vi "Read_Input_1.vi"(8 "Error_In":errorcluster, 11 "Calculator_In":refnum<class "Calculator.lvclass">) -> (0 "Error_Out":errorcluster, 2 "Input_1":dbl, 3 "Calculator_Out":refnum<class "Calculator.lvclass">)   [LabVIEW 2021, in "Calculator.lvclass"]
doc: "Used to read the data of input 1 of calculator class"
uses:
  Calculator.lvclass
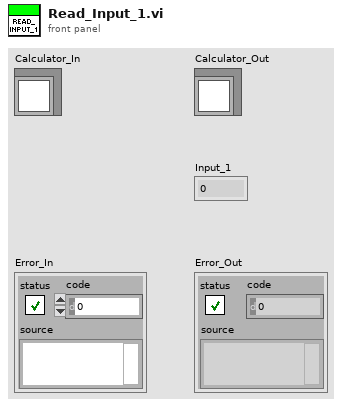
[diagram p1: front panel]
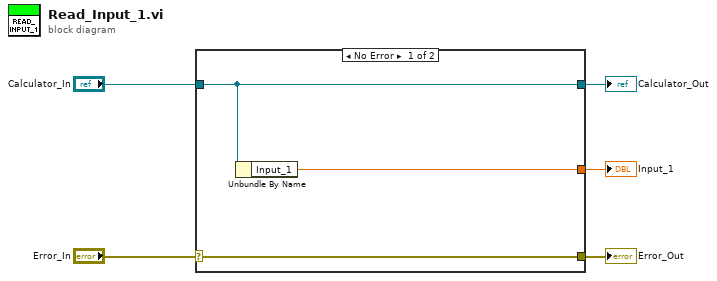
[diagram p0: block diagram]
diagram:
  n1 = case shown="No Error" "Error_In" {
    selector: "Error_In" -> [w8 w9]
    tunnel: [w8 w9] -> w4
    tunnel: [w7 w10] -> w2
    tunnel: "Calculator_In" -> [w7 w10]
    tunnel: [w6 _] -> w1
    frame No Error {
      n2 = Unbundle By Name(w7) -> ("Input_1"=w6:dbl)
    }
    frame Error {
    }
  }
  "Error_Out" <- w4
  "Calculator_Out" <- w2
  "Input_1" <- w1
